vi "Standard Setup.vi"(8 "error in (no error)":errorcluster, 11 "CCDCamera in":refnum<class "Simulated_CCD_Camera.lvclass">) -> (0 "error out":errorcluster, 3 "CCDCamera out":refnum<class "Simulated_CCD_Camera.lvclass">)   [LabVIEW 2018, in "Simulated_CCD_Camera.lvclass"]
uses:
  Simulated_CCD_Camera.lvclass
  <userlib>/atmcd32d.llb/HSSpeed_type typedef.ctl
  <userlib>/atmcd32d.llb/Shutter_mode typedef.ctl
  Simulated_CCD_Camera.lvclass/Simulated_CCD_Camera.ctl
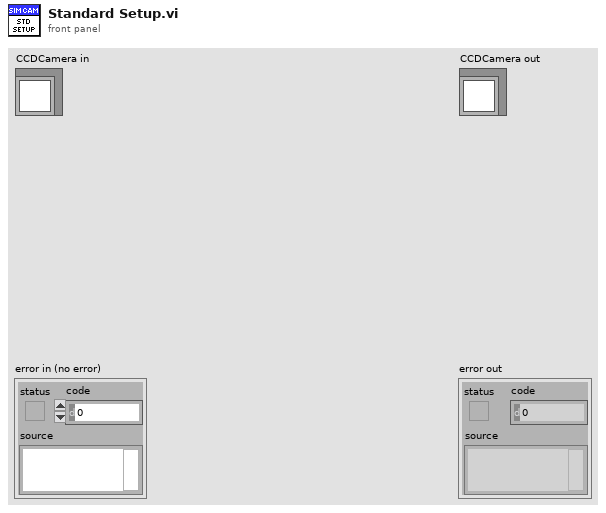
[diagram p1: front panel]
types:
  T1 = typedef "Shutter_mode typedef.ctl" = enum16{"Auto", "Open", "Close", "N/A (3)", "Open FVB Series", "Open Any Series"}
  T2 = typedef "HSSpeed_type typedef.ctl" = enum16{"EM Amp", "Conventional Amp"}
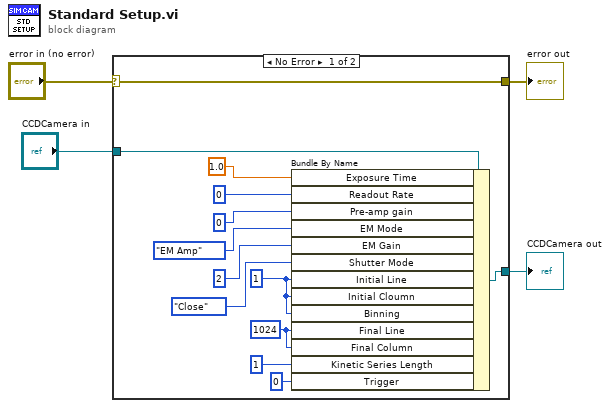
[diagram p0: block diagram]
diagram:
  n1 = case shown="No Error" "error in (no error)" {
    selector: "error in (no error)" -> [w17 w19]
    tunnel: [w17 w19] -> w2
    tunnel: [w15 w18] -> w1
    tunnel: "CCDCamera in" -> [w16 w18]
    frame No Error {
      w7 = u16 1024 ("Initial Line")
      w8 = u16 1 ("Initial Line")
      n2 = Bundle By Name(cluster=w16, "Exposure Time"=1.0, "Readout Rate"=u8 0, "Pre-amp gain"=u8 0, "EM Mode"=HSSpeed_type_typedef."EM Amp" ("type"), "EM Gain"=u16 2, "Shutter Mode"=Shutter_mode_typedef."Close" ("mode"), "Initial Line"=w8, "Initial Cloumn"=w8, "Binning"=w8, "Final Line"=w7, "Final Column"=w7, "Kinetic Series Length"=1, "Trigger"=u16 0 ("CCD Config.Trigger")) -> (w15:refnum<class "Simulated_CCD_Camera.lvclass">)
    }
    frame Error {
    }
  }
  "error out" <- w2
  "CCDCamera out" <- w1
